vi "initialize.vi"(8 "error in (no error)":errorcluster, 11 "instrument in":refnum<class "instrument.lvclass">) -> (0 "error out":errorcluster, 1 "String outout":string, 2 "initialized?":bool, 3 "instrument out":refnum<class "instrument.lvclass">)   [LabVIEW 2017, in "instrument.lvclass"]
doc: "initializes an instrument; this method is going to be replaced by the same method of the child objects"
uses:
  instrument.lvclass
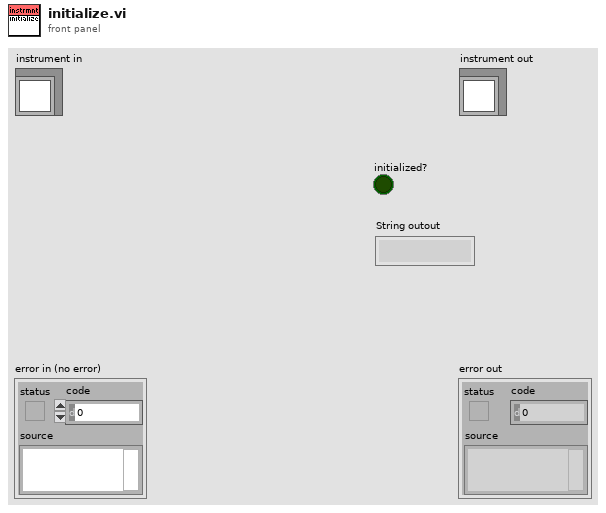
[diagram p1: front panel]
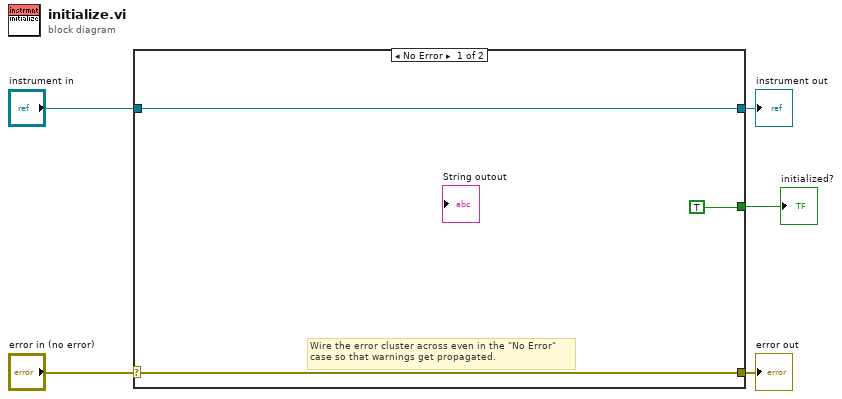
[diagram p0: block diagram]
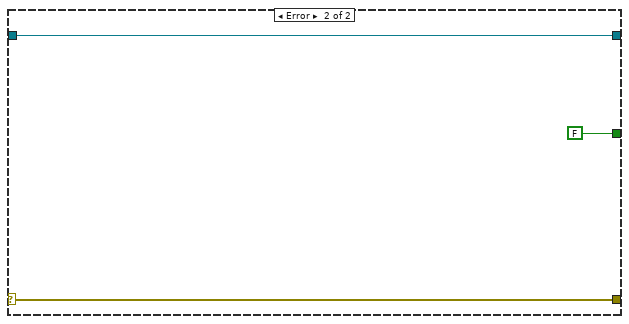
[diagram p2: hidden frame]
diagram:
  n1 = case shown="No Error" "error in (no error)" {
    selector: "error in (no error)" -> [w7 w11]
    tunnel: [w7 w11] -> w4
    tunnel: [w8 w10] -> w2
    tunnel: "instrument in" -> [w8 w10]
    tunnel: [TRUE ("initialized?") FALSE ("initialized?")] -> w1
    frame No Error {
      # "Wire the error cluster across even in the \"No Error\"\ncase so that warnings get propagated."
    }
    frame Error {
    }
  }
  "error out" <- w4
  "instrument out" <- w2
  "initialized?" <- w1
